vi "main_test.vi"   [LabVIEW 2015]
uses:
  GOD.lvclass
  General.lvclass
  A/A.lvclass
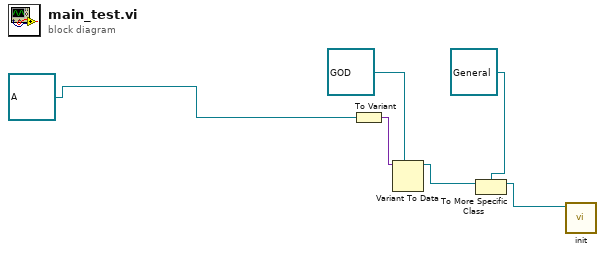
[diagram p0: block diagram]
diagram:
  n1 = To Variant(anything=refnum<class "A.lvclass"> refnum ("A.lvclass")) -> (Variant=w6:variant)
  n2 = Variant To Data(type=refnum<class "GOD.lvclass"> refnum ("GOD.lvclass"), Variant=w6) -> (data=w4:refnum<class "GOD.lvclass">)  [unwired: 1 in, 1 out]
  n3 = To More Specific Class(target class=refnum<class "General.lvclass"> refnum ("General.lvclass"), reference=w4) -> (specific class reference=w2:refnum<class "General.lvclass">)  [unwired: 1 in, 1 out]
  n4 = call-dynamic "init.vi"("General in"=w2) -> ()  [unwired: 9 in, 2 out]
